vi "Handle error.vi"(8 "error in (no error)":T1, 10 "module loopdata":T2) -> ()   [LabVIEW 2019, in "ModuleTemplate.lvlib"]
doc: "Handles error occured in module.\nProvides additional error info and triggers \"Error\" event\nDecides next module state"
uses:
  ModuleTemplate.lvlib
  module data.ctl
  SubVIs/Shared/Shared.lvlib
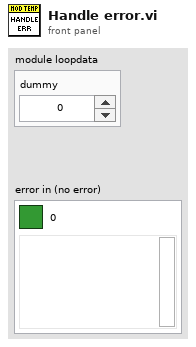
[diagram p1: front panel]
types:
  T1 = cluster{"Boolean Round":bool, "code":i32, "source":string}
  T2 = typedef "ModuleTemplate.lvlib/module data.ctl" = cluster{"dummy":dbl}
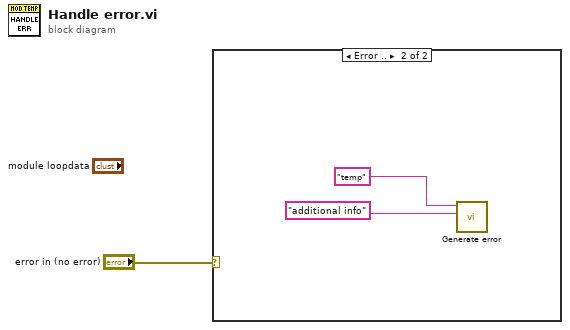
[diagram p0: block diagram]
diagram:
  n1 = case shown="Error .." "error in (no error)" {
    frame No Error {
    }
    frame Error {
      n2 = call "Generate error.vi"("info"="additional info" ("module"), "module"="temp") -> ()  [unwired: 9 in, 1 out]
    }
  }
